vi "Drive Problem Fix.vi"(1 "Drive Info Modified":T1, 2 "Drive Info Original":T1) -> (0 "Drive Info Fixed":T1)   [LabVIEW 2013]
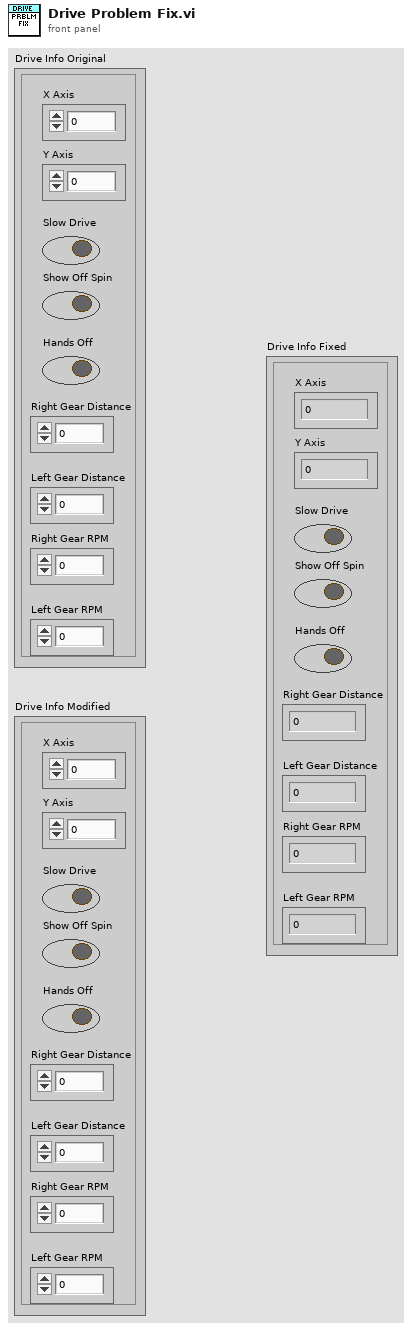
[diagram p1: front panel]
types:
  T1 = cluster{"X Axis":dbl, "Y Axis":dbl, "Slow Drive":bool, "Show Off Spin":bool, "Hands Off":bool, "Right Gear Distance":dbl, "Left Gear Distance ":dbl, "Right Gear RPM":dbl, "Left Gear RPM":dbl}
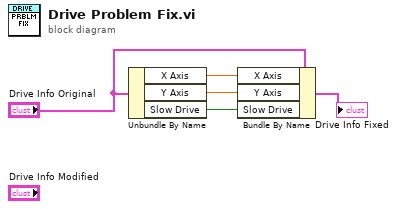
[diagram p0: block diagram]
diagram:
  n1 = Unbundle By Name("Drive Info Original") -> ("X Axis"=w3:dbl, "Y Axis"=w2:dbl, "Slow Drive"=w1:bool)
  n2 = Bundle By Name(cluster="Drive Info Original", "X Axis"=w3, "Y Axis"=w2, "Slow Drive"=w1) -> (→"Drive Info Fixed":T1)
